vi "Local Configuration.INTCSR.Local DMA Interrupt Enable.Get.vi"(8 "error in (no error)":errorcluster, 11 "GE 5565PIORC":refnum<class "GE 5565PIORC.lvclass">) -> (0 "error out":errorcluster, 2 "Local DMA Interrupt Enabled?":bool, 3 "GE 5565PIORC out":refnum<class "GE 5565PIORC.lvclass">)   [LabVIEW 2016, in "GE 5565PIORC.lvclass"]
uses:
  GE 5565PIORC.lvclass
  Controls/Registers.Local Configuration.ctl
  GE 5565PIORC.lvclass/GE 5565PIORC.ctl
  <vilib>/Instr/_visa.llb/VISA Register Access Address Space.ctl
  Binary Operations/Get Bits U32.vi
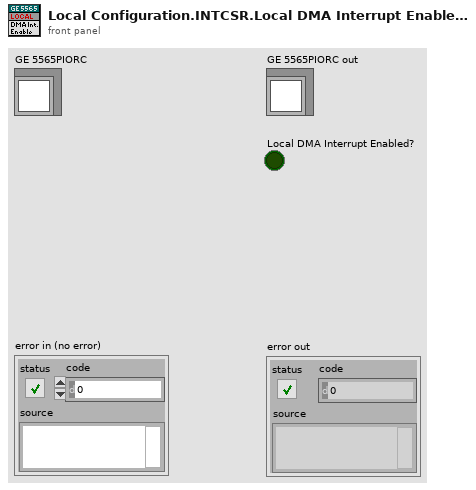
[diagram p1: front panel]
types:
  T1 = typedef "GE 5565PIORC.lvclass/Registers.Local Configuration.ctl" = enum16{"DMA Arbitration", "Interrupt Control and Status", "DMA Mode", "DMA PCI Address", "DMA Local Address", "DMA Transfer Size", "DMA Descriptor Pointer", "DMA Command/Status", "DMA PCI DAC Upper Address", "PCI PIO Address Range", "PCI PIO Base Address (Remap)"}
  T2 = typedef "VISA Register Access Address Space.ctl" = u16
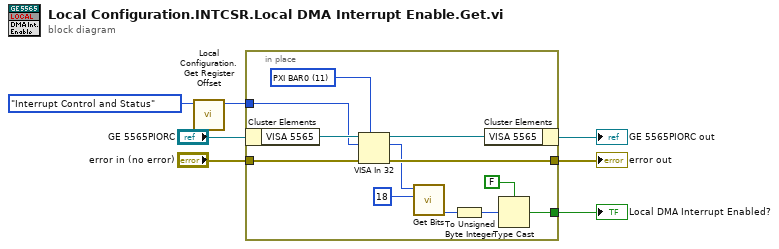
[diagram p0: block diagram]
diagram:
  n1 = call "Local Configuration.Get Register Offset.vi"("Local Configuration Register"=Registers.Local_Configuration."Interrupt Control and Status" ("Local Configration Register Offset")) -> ("Offset"=w1:u32)  [unwired: 10 in]
  n2 = in-place {
    in-place-border: "error in (no error)" -> [w17]
    in-place-border: [w16] -> w5
    in-place-border: [w9] -> w3
    in-place-border: w1 -> [w8]
    w13 = T2 11 items=["VXI/VME A16"=1, "VXI/VME A24"=2, "VXI/VME A32"=3, "VXI/VME A64"=4, "PXI Memory Allocations"=9, "PXI Configuration"=10, "PXI BAR0"=11, "PXI BAR1"=12, "PXI BAR2"=13, "PXI BAR3"=14, "PXI BAR4"=15, "PXI BAR5"=16] ("Address Space")
    n3 = in-place-cluster #1("GE 5565PIORC") -> ("VISA 5565"=w19:refnum<visa-resource-name>)
    n4 = VISA In 32(7:w13, 8:w17, 10:w8, 11:w19) -> (0:w16:errorcluster, 2:w15:u32, 3:w18:refnum<visa-resource-name>)
    n5 = call-poly "Get Bits.vi"("Start Index (0)"=u8 18, "Register in"=w15) -> ("Value"=w12:u32)  [unwired: 6 in, 3 out]
    n6 = To Unsigned Byte Integer(number=w12) -> (unsigned 8bit integer=w11:u8)
    n7 = in-place-cluster #1("VISA 5565"=w18) -> (→"GE 5565PIORC out":refnum<class "GE 5565PIORC.lvclass">)
    n8 = Type Cast(type=FALSE, x=w11) -> (*(type *) &x=w9:bool)
  }
  "error out" <- w5
  "Local DMA Interrupt Enabled?" <- w3
